vi "Pre-Build Action.vi"(6 "Top Level/Always Included VIs":path[](array[path]), 7 "Main Destination Path":path, 9 "Target Name":string, 10 "Build Specification Name":string, 11 "Project Path":path) -> (0 "error out":errorcluster)   [LabVIEW 2024, in "Launcher Support.lvlib"]
doc: "This Pre-Build Action VI sets the Debug mode to false to ensure the top level VI has the headless properties at build time.\n_____\nBased on DQMH Dev Tools: Project Template 7.1.0.1503."
uses:
  Launcher Support.lvlib
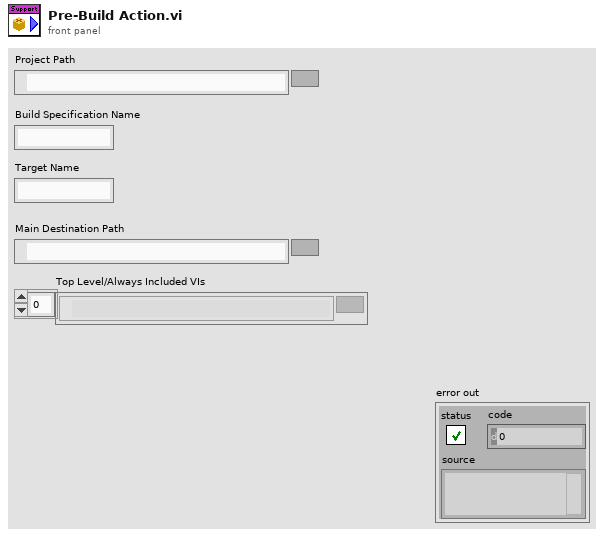
[diagram p1: front panel]
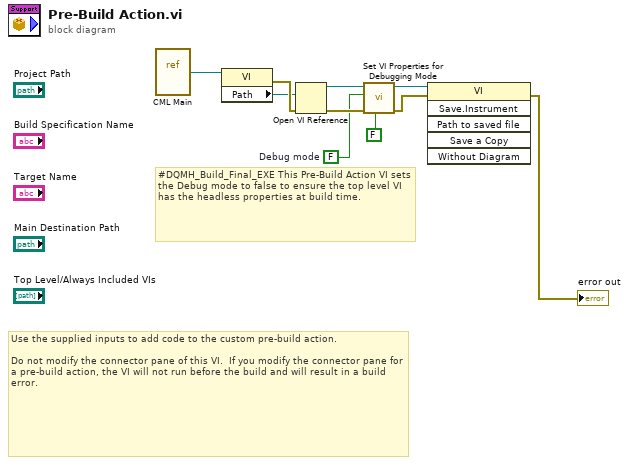
[diagram p0: block diagram]
diagram:
  w5 = FALSE  # Debug mode
  # "#DQMH_Build_Final_EXE This Pre-Build Action VI sets the Debug mode to false to ensure the top level VI has the headless properties at build time."
  # "Use the supplied inputs to add code to the custom pre-build action.\n\nDo not modify the connector pane of this VI.  If you modify the connector pane for a pre-build action, the VI will not run before the build and will result in a build error."
  n1 = vi-ref "CML Main.vi"() -> (w8:refnum<vi>)
  n2 = property class="VI"(reference=w8) -> (error out=w10:errorcluster, "Path"=w7:path)  [unwired: 1 in, 1 out]
  n3 = Open VI Reference(vi path=w7, error in (no error)=w10) -> (vi reference=w6:refnum<vi>, error out=w9:errorcluster)  [unwired: 4 in]
  n4 = call "Set VI Properties for Debugging Mode.vi"("Red?"=FALSE, "error in"=w9, "Debug mode?"=w5, "Launcher VI ref"=w6) -> ("error out"=w2:errorcluster, "Launcher VI ref out"=w4:refnum<vi>)  [unwired: 6 in]
  n5 = invoke class="VI" method="Save.Instrument"(reference=w4, error in=w2) -> (error out=→"error out":errorcluster)  [unwired: 4 in, 5 out]
